vi "SetFailedIconToSubtree.vi"(8 "error in (no error)":errorcluster, 10 "Active Parent":string, 11 "ResultTree in":refnum<class "ResultTree.lvclass">) -> (0 "error out":errorcluster, 3 "ResultTree out":refnum<class "ResultTree.lvclass">)   [LabVIEW 2019, in "ResultTreeListener.lvclass"]
uses:
  ResultTreeListener.lvclass
  ResultTree/ResultTree.lvclass
  ResultTree/Icon.ctl
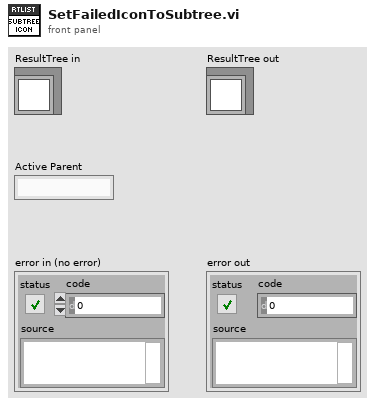
[diagram p1: front panel]
types:
  T1 = typedef "ResultTree.lvclass/Icon.ctl" = enum16{"None", "Passed", "Failed", "Error"}
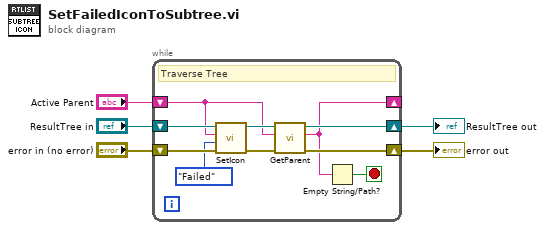
[diagram p0: block diagram]
diagram:
  n1 = while {
    shift-right: [w10] -> w3
    shift-left: "ResultTree in" -> [w15]
    shift-right: [w9] -> w2
    shift-left: "error in (no error)" -> [w14]
    shift-right: [w7] -> _
    shift-left: "Active Parent" -> [w11]
    stop <- w6 stop-if-true
    # "Traverse Tree"
    n2 = call "SetIcon.vi"("error in (no error)"=w14, "Icon"=Icon."Failed", "Tag Name"=w11, "ResultTree in"=w15) -> ("error out"=w12:errorcluster, "ResultTree out"=w13:refnum<class "ResultTree.lvclass">)  [unwired: 6 in]
    n3 = call "GetParent.vi"("error in (no error)"=w12, "Tag"=w11, "ResultTree in"=w13) -> ("error out"=w9:errorcluster, "Parent Tag"=w7:string, "ResultTree out"=w10:refnum<class "ResultTree.lvclass">)  [unwired: 6 in]
    n4 = Empty String/Path?(string/path=w7) -> (empty?=w6:bool)
  }
  "ResultTree out" <- w3
  "error out" <- w2
